vi "Initialize New Category Display.vi"(8 "error in (no error)":errorcluster, 10 "Name to Display":string, 11 "Configuration in":refnum<class "Configuration.lvclass">) -> (0 "error out":errorcluster, 2 "Change Display":refnum<user-event>, 3 "Configuration Out":refnum<class "Configuration.lvclass">)   [LabVIEW 2016, in "Configuration.lvlib" / "Configuration.lvclass"]
uses:
  <userlib>/Configuration Dialog Actor/Configuration.lvclass
  <userlib>/Configuration Dialog Actor/Configuration.lvclass/Configuration.ctl
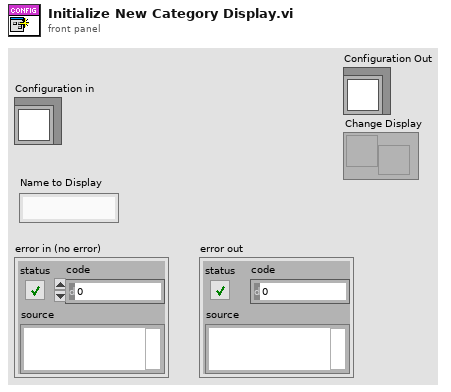
[diagram p1: front panel]
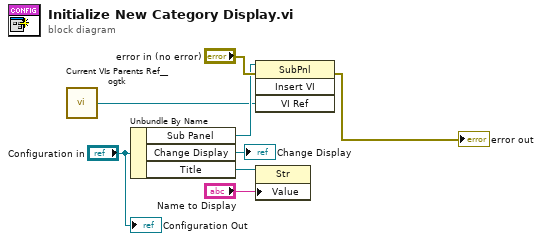
[diagram p0: block diagram]
diagram:
  n1 = call <userlib>:"Current VIs Parents Ref__ogtk.vi"() -> ("Calling VI's Reference"=w4:refnum<vi>)  [unwired: 2 in]
  n2 = Unbundle By Name("Configuration in") -> ("Sub Panel"=w6:refnum<vi>, "Change Display"=→"Change Display":refnum<user-event>, "Title"=w3:refnum<vi>)
  n3 = invoke class="SubPnl" method="Insert VI"(reference=w6, error in="error in (no error)", "VI Ref"=w4) -> (error out=→"error out":errorcluster)  [unwired: 1 in, 3 out]
  n4 = property class="Str"(reference=w3, "Value"="Name to Display") -> ()  [unwired: 1 in, 2 out]
  "Configuration Out" <- "Configuration in"
